vi "IIC Write Bytes Of Event.vi"(1 "TimeOutOfEventMs":i32, 4 "EventType":u8, 5 "EventPin":i32, 6 "WriteLen":i32, 7 "pWriteData":u8, 9 "SlaveAddr":i16, 10 "IICIndex":i32, 11 "DevHandle":i32) -> (2 "function return":i32, 3 "pWriteData out":u8)   [LabVIEW 2010, in "usb2iic.lvlib"]
doc: "int WINAPI IIC_WriteBytesOfEvent(int DevHandle,int IICIndex,short SlaveAddr,unsigned char *pWriteData,int WriteLen,int EventPin,unsigned char EventType,int TimeOutOfEventMs);"
uses:
  usb2iic.lvlib
  USB2XXX.dll
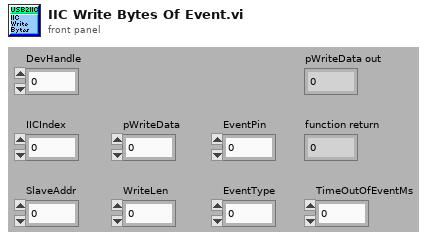
[diagram p1: front panel]
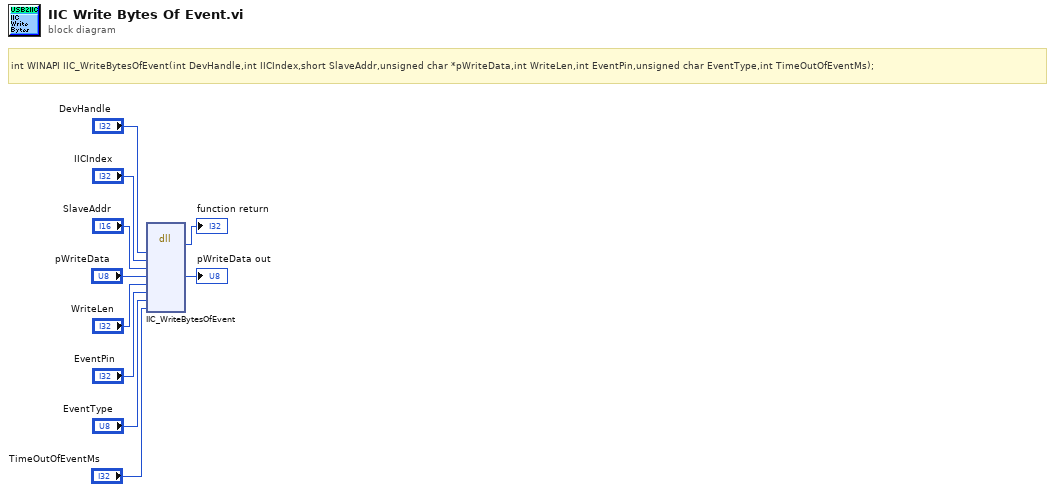
[diagram p0: block diagram]
diagram:
  # "int WINAPI IIC_WriteBytesOfEvent(int DevHandle,int IICIndex,short SlaveAddr,unsigned char *pWriteData,int WriteLen,int EventPin,unsigned char EventType,int TimeOutOfEventMs);"
  n1 = dll-call lib="G:/OtherWork/USB2XXX_Example/trunk/Labview/PublicFiles/usb2iic/USB2XXX.*" fn="IIC_WriteBytesOfEvent"("DevHandle"="DevHandle", "IICIndex"="IICIndex", "SlaveAddr"="SlaveAddr", "pWriteData"="pWriteData", "WriteLen"="WriteLen", "EventPin"="EventPin", "EventType"="EventType", "TimeOutOfEventMs"="TimeOutOfEventMs") -> (→"function return":i32, "pWriteData"=→"pWriteData out":u8)  [unwired: 10 in, 2 out]
